vi "Timed Message-Core_Process.vi"(0 "FTW Actor Instance Configuration":string="{\n  \"Identity\": \"ActorName\",\n  \"InboxAddress\": \"tcp://127.0.0.1:*\",\n  \"PublisherAddress\": \"tcp://127.0.0.1:*\",\n  \"DebugEnableInboxLogging\": false,\n  \"DebugEnableJobLogging\": false,\n  \"DebugShowPanel\": false\n}", 11 "ErrorIn":errorcluster) -> (15 "Error":errorcluster)   [LabVIEW 2012, in "Timed Message-Core.lvclass"]
uses:
  Timed Message-Core.lvclass
  Timed Message-Core.lvclass/Timed Message-Core.ctl
  src/Connector/FTW-ActorConnector.lvclass
  Core/src/Time/FTW-Time-DisplayFormat-Timestamp.ctl
  src/Instance/FTW-ActorInstance.lvclass
  src/Message/Request/FTW-Message-IncomingRequest.lvclass
panel:
  # "#TODO\nhide controls for a GUI"
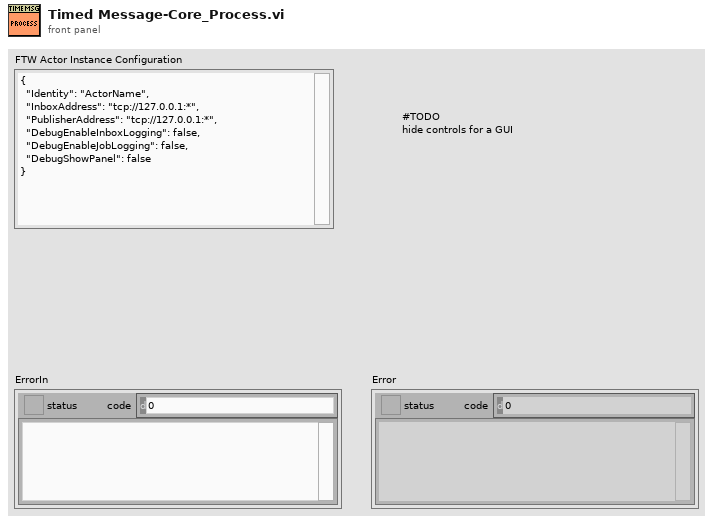
[diagram p1: front panel]
types:
  T1 = typedef "FTW-Time-DisplayFormat-Timestamp.ctl" = enum16{"YYYY-MM-DDT00:00:00.000Z (ISO-8601)", "YYYY-MM-DDT00-00-00Z (Simple ISO-8601)", "YYYY-MM-DD"}
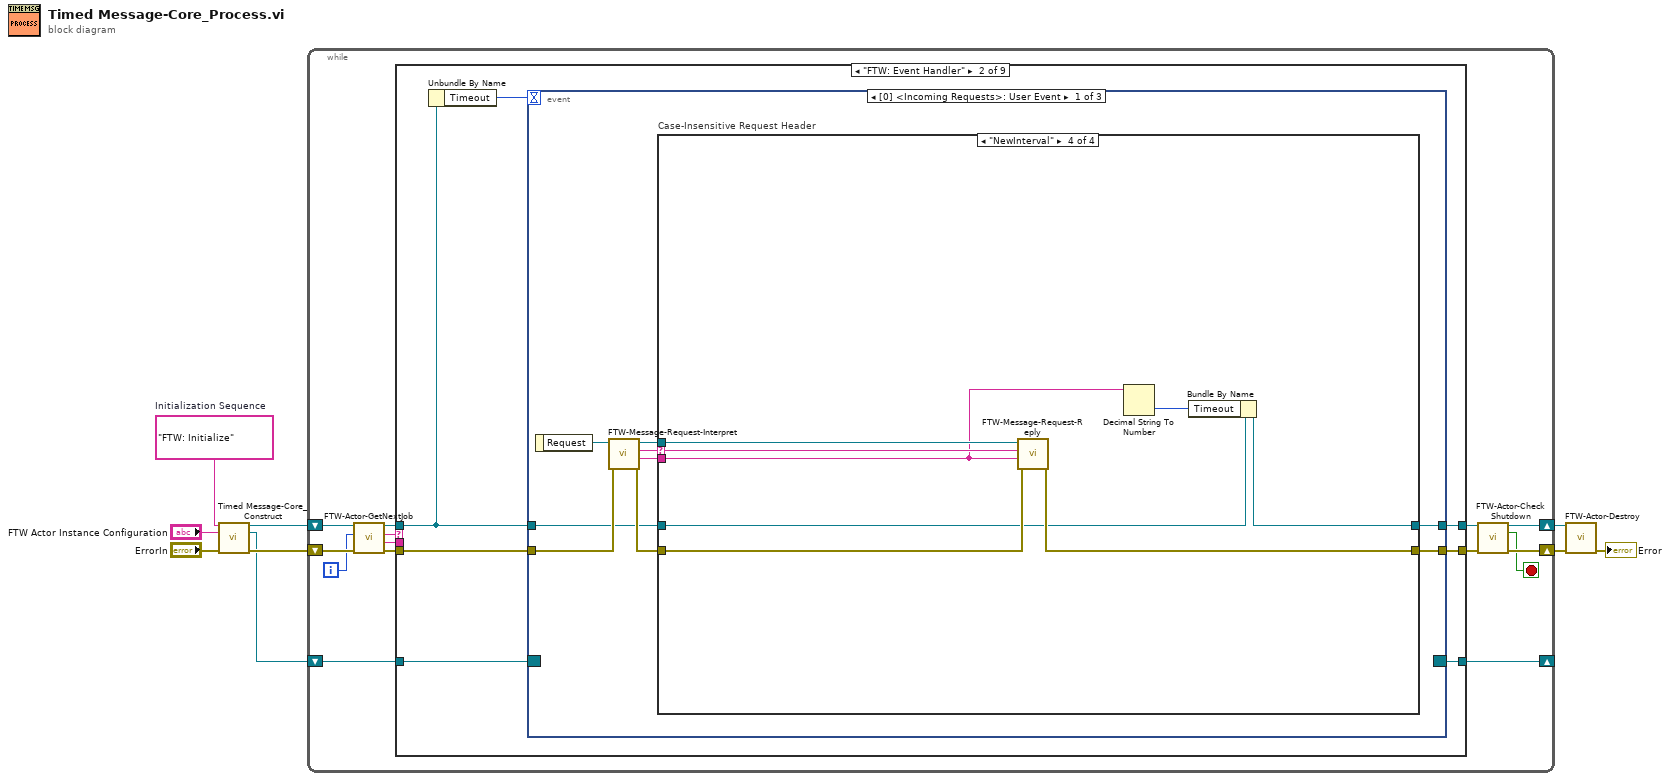
[diagram p0: block diagram]
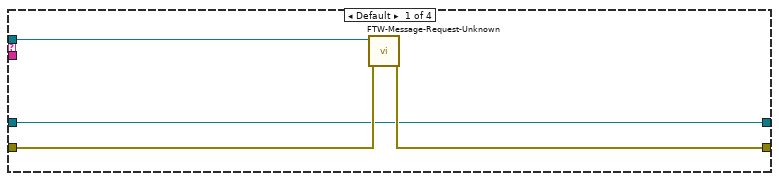
[diagram p3: hidden frame]
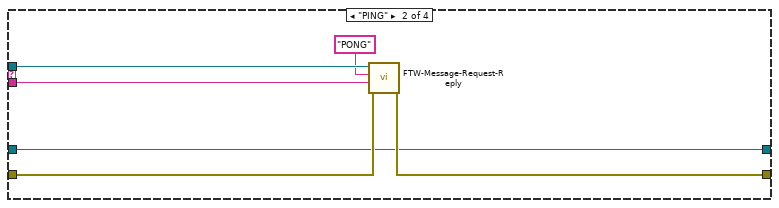
[diagram p4: hidden frame]
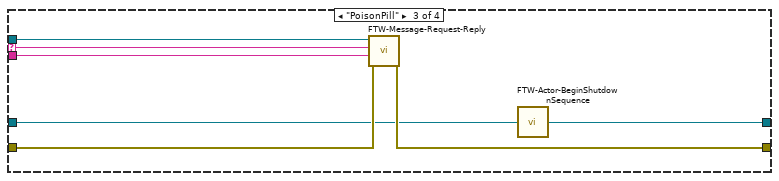
[diagram p5: hidden frame]
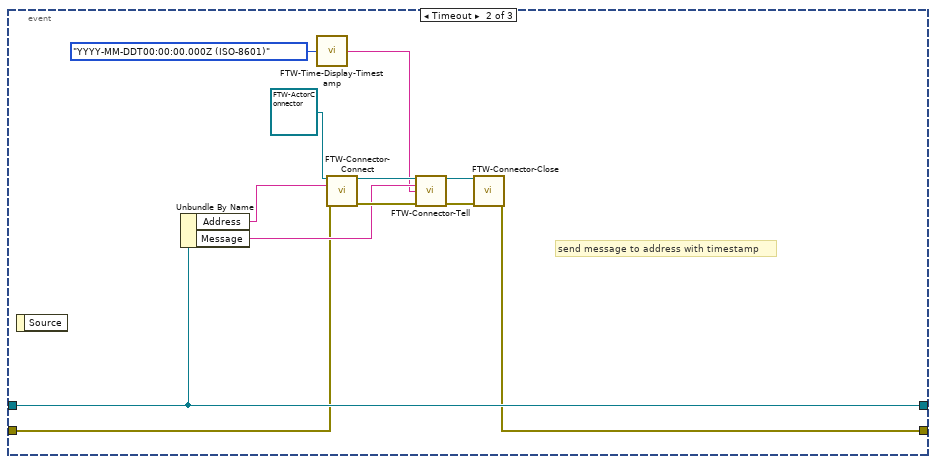
[diagram p6: hidden frame]
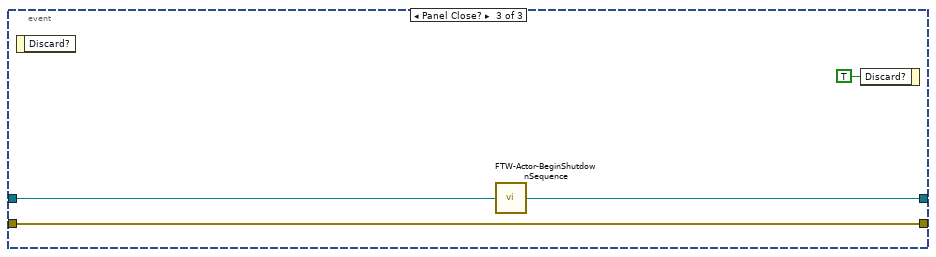
[diagram p7: hidden frame]
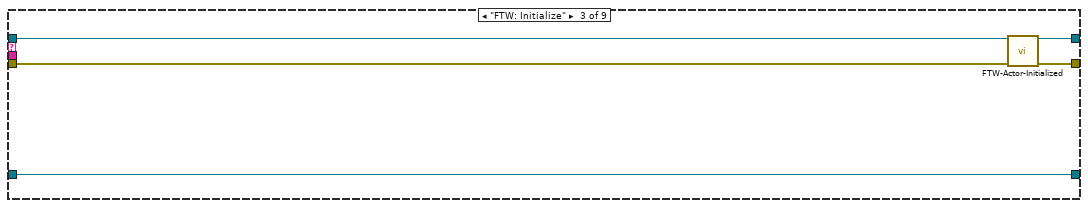
[diagram p8: hidden frame]
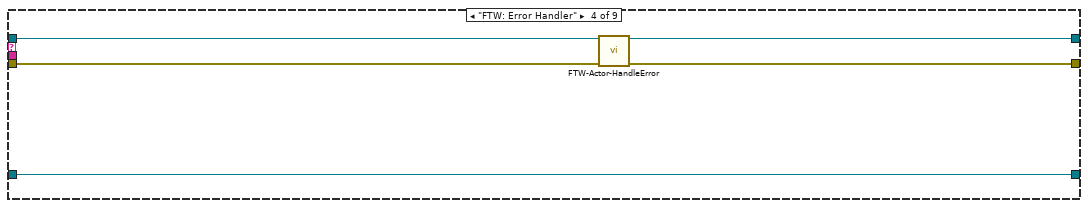
[diagram p9: hidden frame]
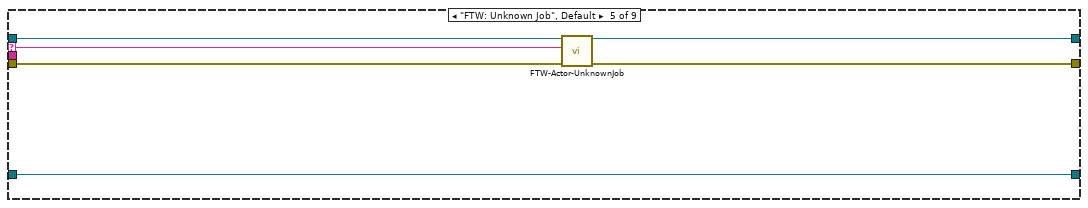
[diagram p10: hidden frame]
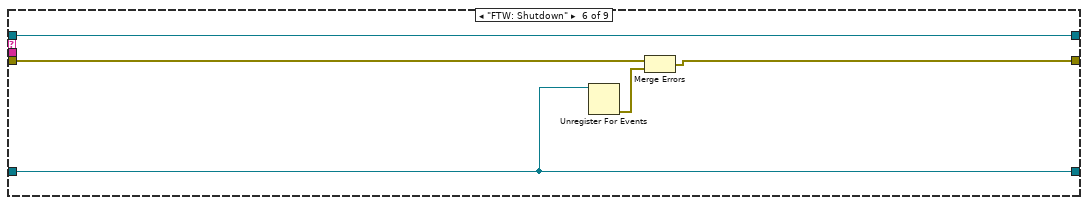
[diagram p11: hidden frame]
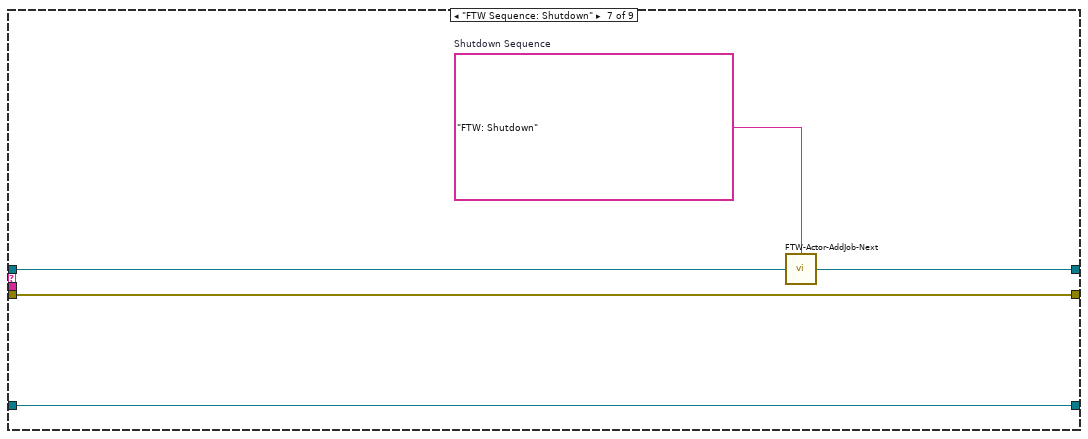
[diagram p12: hidden frame]
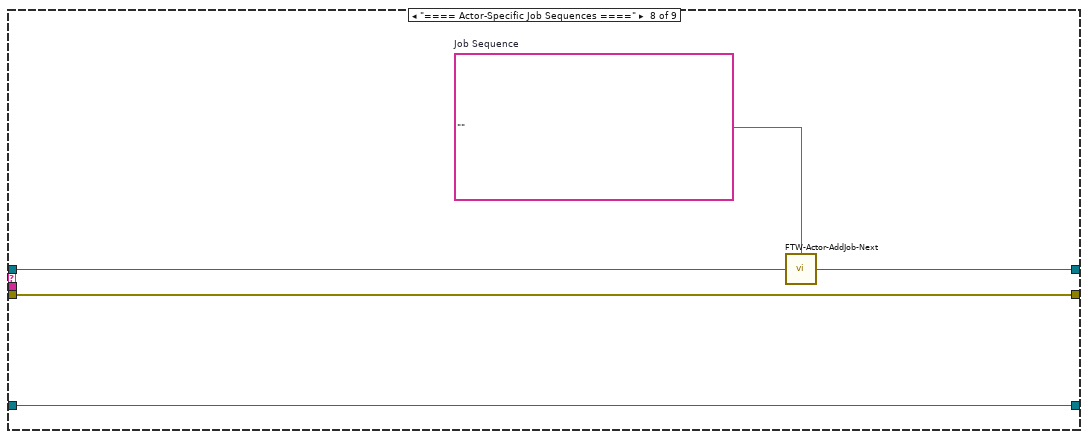
[diagram p13: hidden frame]
diagram:
  w4 = "FTW: Initialize"  # Initialization Sequence
  n1 = call "Timed Message-Core_Construct.vi"("Initialization Sequence"=w4, "FTW Actor Instance Configuration"="FTW Actor Instance Configuration", "error in (no error)"="ErrorIn") -> ("Timed Message-Core out"=w9:refnum<class "Timed Message-Core.lvclass">, "Incoming Requests"=w1:refnum<event-registration>, "error out"=w5:errorcluster)  [unwired: 10 in]
  n2 = while {
    shift-right: [w13] -> w7
    shift-left: w5 -> [w20]
    shift-right: [w10] -> _
    shift-left: w1 -> [w23]
    shift-right: [w15] -> w8
    shift-left: w9 -> [w22]
    i -> [w11]
    stop <- w12 stop-if-true
    n3 = call "FTW-Actor-GetNextJob.vi"("error in"=w20, "Jobs Performed"=w11, "FTW Actor Instance"=w22) -> ("error out"=w19:errorcluster, "Job Data"=w17:string, "Job Name"=w18:string, "FTW Actor Instance out"=w21:refnum<class "Timed Message-Core.lvclass">)  [unwired: 5 in]
    n4 = case shown="\"FTW: Event Handler\"" w18 {
      selector: w18 -> [_ _ _ _ w94 _ _ _ _]
      tunnel: [w25 w33 w84 w89 w97 w103 w108 w113 w117] -> w14
      tunnel: w19 -> [w25 w32 w87 w91 w98 w104 w108 w113 w117]
      tunnel: w23 -> [w26 w29 w88 w93 w99 w100 w109 w114 w116]
      tunnel: [w26 w31 w88 w93 w99 w100 w109 w114 w116] -> w10
      tunnel: w17 -> [_ _ _ _ _ _ _ _ _]
      tunnel: [w24 w30 w85 w90 w95 w101 w106 w111 w115] -> w16
      tunnel: w21 -> [w24 w28 w86 w92 w96 w101 w107 w112 w115]
      frame "==== Featherweight Framework Jobs ====" {
      }
      frame "FTW: Event Handler" {
        n5 = Unbundle By Name(w28) -> ("Timeout"=w27:i32)
        n6 = event shown="[0] <Incoming Requests>: User Event" {
          selector: w29 -> [_ _ _]
          dyn-events: [_ _ _] -> w31
          timeout: w27 -> [_ _ _]
          tunnel: [w39 w70 w82] -> w33
          tunnel: w32 -> [w40 w71 w82]
          tunnel: [w38 w78 w80] -> w30
          tunnel: w28 -> [w37 w78 w81]
          event User Event {
            n7 = event-data() -> ("Request"=w41:refnum<class "FTW-Message-IncomingRequest.lvclass">)  [unwired: 1 in]
            n8 = call "FTW-Message-Request-Interpret.vi"("error in"=w40, "FTW Incoming Request"=w41) -> ("error out"=w42:errorcluster, "Request Body"=w35:string, "Request Header"=w36:string, "FTW Incoming Request out"=w34:refnum<class "FTW-Message-IncomingRequest.lvclass">)  [unwired: 6 in]
            n9 = case "Case-Insensitive Request Header" shown="\"NewInterval\"" w36 {
              selector: w36 -> [_ _ w54 w63]
              tunnel: [w45 w49 w56 w65] -> w39
              tunnel: w42 -> [w46 w50 w57 w66]
              tunnel: [w43 w47 w59 w62] -> w38
              tunnel: w37 -> [w43 w47 w55 w64]
              tunnel: w35 -> [_ w51 w53 w60]
              tunnel: w34 -> [w44 w52 w58 w67]
              frame Default {
                n10 = call "FTW-Message-Request-Unknown.vi"("error in"=w46, "FTW Incoming Request"=w44) -> ("error out"=w45:errorcluster)  [unwired: 9 in]
              }
              frame "PING" {
                n11 = call "FTW-Message-Request-Reply.vi"("error in"=w50, "Response Body"=w51, "Response Header"="PONG", "FTW Incoming Request"=w52) -> ("error out"=w49:errorcluster)  [unwired: 6 in, 1 out]
              }
              frame "PoisonPill" {
                n12 = call "FTW-Message-Request-Reply.vi"("error in"=w57, "Response Body"=w53, "Response Header"=w54, "FTW Incoming Request"=w58) -> ("error out"=w56:errorcluster)  [unwired: 6 in, 1 out]
                n13 = call "FTW-Actor-BeginShutdownSequence.vi"("FTW Actor Instance"=w55) -> ("FTW Actor Instance out"=w59:refnum<class "Timed Message-Core.lvclass">)  [unwired: 3 in]
              }
              frame "NewInterval" {
                n14 = call "FTW-Message-Request-Reply.vi"("error in"=w66, "Response Body"=w60, "Response Header"=w63, "FTW Incoming Request"=w67) -> ("error out"=w65:errorcluster)  [unwired: 6 in, 1 out]
                n15 = Decimal String To Number(string=w60) -> (number=w61:i32)  [unwired: 2 in, 1 out]
                n16 = Bundle By Name(cluster=w64, "Timeout"=w61) -> (w62:refnum<class "Timed Message-Core.lvclass">)
              }
            }
          }
          event Timeout {
            # "send message to address with timestamp"
            n17 = event-data() -> ()  [unwired: 1 in, 1 out]
            n18 = Unbundle By Name(w78) -> ("Address"=w77:string, "Message"=w74:string)
            n19 = call "FTW-Time-Display-Timestamp.vi"("Format"=FTW-Time-DisplayFormat-Timestamp."YYYY-MM-DDT00:00:00.000Z (ISO-8601)") -> ("Formatted Timestamp"=w68:string)  [unwired: 3 in]
            n20 = call-dynamic "FTW-Connector-Connect.vi"("FTW Actor Connector Type"=refnum<class "FTW-ActorConnector.lvclass"> refnum, "Instance Inbox Address"=w77, "error in"=w71) -> ("FTW Actor Connector"=w76:refnum<class "FTW-ActorConnector.lvclass">, "error out"=w75:errorcluster)  [unwired: 11 in]
            n21 = call "FTW-Connector-Tell.vi"("FTW Actor Connector"=w76, "Message Header"=w74, "Message Body"=w68, "error in"=w75) -> ("FTW Actor Connector out"=w73:refnum<class "FTW-ActorConnector.lvclass">, "error out"=w72:errorcluster)  [unwired: 9 in, 1 out]
            n22 = call-dynamic "FTW-Connector-Close.vi"("FTW Actor Connector"=w73, "error in"=w72) -> ("error out"=w70:errorcluster)  [unwired: 13 in]
          }
          event Panel Close? {
            n23 = event-data() -> ()  [unwired: 1 in, 1 out]
            n24 = call "FTW-Actor-BeginShutdownSequence.vi"("FTW Actor Instance"=w81) -> ("FTW Actor Instance out"=w80:refnum<class "Timed Message-Core.lvclass">)  [unwired: 3 in]
            n25 = event-data("Discard?"=TRUE) -> ()  [unwired: 1 in, 1 out]
          }
        }
      }
      frame "FTW: Initialize" {
        n26 = call-dynamic "FTW-Actor-Initialized.vi"("FTW Actor Instance"=w86, "error in"=w87) -> ("FTW Actor Instance out"=w85:refnum<class "Timed Message-Core.lvclass">, "error out"=w84:errorcluster)  [unwired: 12 in]
      }
      frame "FTW: Error Handler" {
        n27 = call-dynamic "FTW-Actor-HandleError.vi"("FTW Actor Instance"=w92, "error in"=w91) -> ("FTW Actor Instance out"=w90:refnum<class "Timed Message-Core.lvclass">, "error out"=w89:errorcluster)  [unwired: 11 in, 1 out]
      }
      frame "FTW: Unknown Job", Default {
        n28 = call-dynamic "FTW-Actor-UnknownJob.vi"("FTW Actor Instance"=w96, "Unknown Job"=w94, "error in"=w98) -> ("FTW Actor Instance out"=w95:refnum<class "Timed Message-Core.lvclass">, "error out"=w97:errorcluster)  [unwired: 11 in]
      }
      frame "FTW: Shutdown" {
        n29 = Unregister For Events(event registration refnum=w100) -> (error out=w102:errorcluster)  [unwired: 1 in]
        n30 = Merge Errors(w104, w102) -> (w103:errorcluster)
      }
      frame "FTW Sequence: Shutdown" {
        w105 = "FTW: Shutdown"  # Shutdown Sequence
        n31 = call "FTW-Actor-AddJob-Next.vi"("Add Next in Job Queue"=w105, "FTW Actor Instance"=w107) -> ("FTW Actor Instance out"=w106:refnum<class "Timed Message-Core.lvclass">)  [unwired: 2 in]
      }
      frame "==== Actor-Specific Job Sequences ====" {
        w110 = ""  # Job Sequence
        n32 = call "FTW-Actor-AddJob-Next.vi"("Add Next in Job Queue"=w110, "FTW Actor Instance"=w112) -> ("FTW Actor Instance out"=w111:refnum<class "Timed Message-Core.lvclass">)  [unwired: 2 in]
      }
      frame "==== Actor-Specific Jobs ====" {
      }
    }
    n33 = call "FTW-Actor-CheckShutdown.vi"("FTW Actor Instance"=w16, "error in"=w14) -> ("FTW Actor Instance out"=w15:refnum<class "Timed Message-Core.lvclass">, "Shutdown?"=w12:bool, "error out"=w13:errorcluster)  [unwired: 11 in]
  }
  n34 = call-dynamic "FTW-Actor-Destroy.vi"("FTW Actor Instance"=w8, "error in"=w7) -> ("error out"=→"Error":errorcluster)  [unwired: 13 in]
